vi "Mock Stop Helper Loop from Process Loop.vi"(8 "error in (no error)":errorcluster, 9 "timeout in ms (-1)":i32, 11 "Mock Process in":refnum<class "Mock Process.lvclass">) -> (0 "error out":errorcluster, 1 "timed out?":bool, 3 "Mock Process out":refnum<class "Mock Process.lvclass">)   [LabVIEW 2020, in "Mock Process.lvclass"]
uses:
  Mock Process.lvclass
  C:/Git/astemes-triarc-framework/source/Framework/Process/Process.lvclass
  Framework/Process/Process.lvclass/Process.ctl
  Framework/Process/Public/Lifecycle/Get Lifecycle State.vi
  Framework/Process/Private/SubVIs/Handle Debug Data.vi
  Framework/Process/Private/SubVIs/Enqueue Request Message.vi
  <vilib>/Utility/error.llb/Clear Errors.vi
  <vilib>/Utility/High Resolution Relative Seconds.vi
  <vilib>/Utility/error.llb/Error Cluster From Error Code.vi
  Framework/Process/Private/SubVIs/Wait for Response Message.vi
  Mock Process.lvclass/Mock Process.ctl
  Framework/Process/Process.lvclass
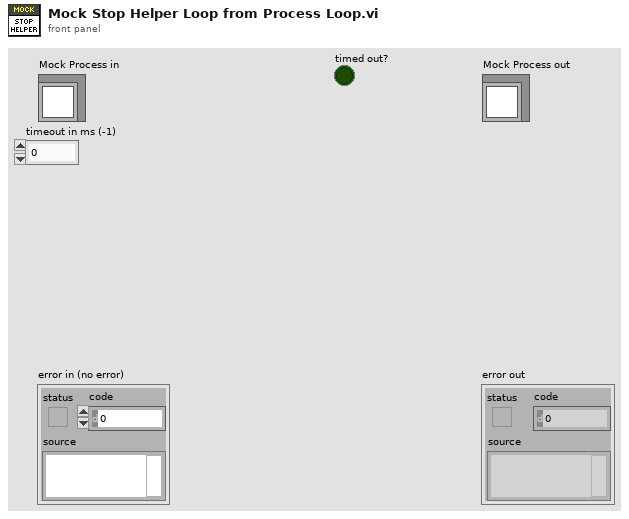
[diagram p1: front panel]
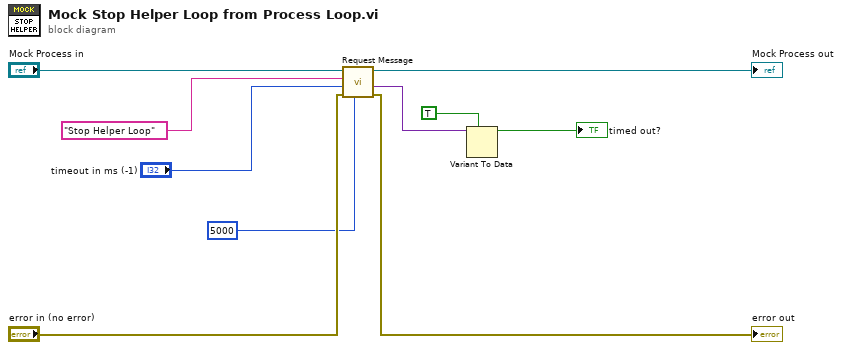
[diagram p0: block diagram]
diagram:
  n1 = call "Request Message.vi"("timeout in ms (-1)"=5000, "error in (no error)"="error in (no error)", "Request Message Data"="timeout in ms (-1)", "Request Message"="Stop Helper Loop", "Process In"="Mock Process in") -> ("error out"=→"error out":errorcluster, "Response Message Data"=w6:variant, "Process Out"=→"Mock Process out":refnum<class "Mock Process.lvclass">)  [unwired: 2 in, 2 out]
  n2 = Variant To Data(type=TRUE, Variant=w6) -> (data=→"timed out?":bool)  [unwired: 1 in, 1 out]
